vi "PSU_Command_Test.vi"() -> ()   [LabVIEW 2020]
uses:
  04db4537-6f8d-454a-96ee-4e1150a41387.vi
  0d439425-5a95-45a5-b8fa-685de4b41df2.vi
panel:
  in  "Stop":bool
  in  "Send":bool
  out "read buffer":string
  out "error out":errorcluster
  in  "write buffer":string
  out "Interface Description":string
  in  "Port":refnum<visa-resource-name>
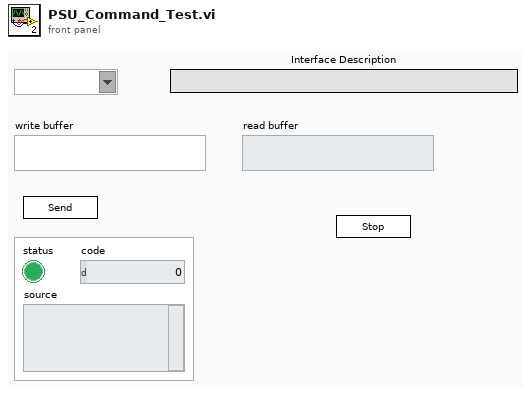
[diagram p1: front panel]
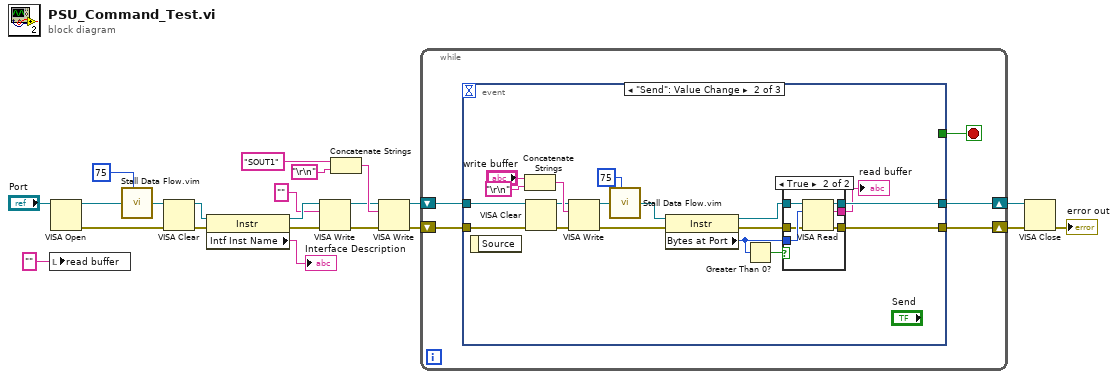
[diagram p0: block diagram]
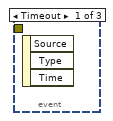
[diagram p2: hidden frame]
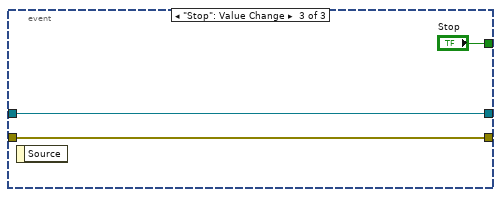
[diagram p4: hidden frame]
diagram:
  n1 = local write "read buffer"("" ("read buffer")) -> ()
  n2 = VISA Open(VISA resource name="Port") -> (VISA resource name=w5:refnum<visa-resource-name>, error out=w6:errorcluster)  [unwired: 4 in]
  n3 = call "Stall Data Flow.vim"("value in"=w5, "milliseconds to wait"=u32 75) -> ("value out"=w4:refnum<visa-resource-name>)  [unwired: 1 out]
  n4 = VISA Clear(VISA resource name=w4, error in (no error)=w6) -> (VISA resource name out=w3:refnum<visa-resource-name>, error out=w2:errorcluster)
  n5 = property class="Instr"(reference=w3, error in=w2) -> (reference out=w12:refnum<visa-resource-name>, error out=w10:errorcluster, "Intf Inst Name"=→"Interface Description":string)
  n6 = VISA Write(VISA resource name=w12, write buffer="", error in (no error)=w10) -> (VISA resource name out=w11:refnum<visa-resource-name>, error out=w9:errorcluster)  [unwired: 1 out]
  n7 = Concatenate Strings("SOUT1" ("string"), "\r\n") -> (w15:string)
  n8 = VISA Write(VISA resource name=w11, write buffer=w15, error in (no error)=w9) -> (VISA resource name out=w13:refnum<visa-resource-name>, error out=w14:errorcluster)  [unwired: 1 out]
  n9 = while {
    shift-right: [w26] -> w18
    shift-left: w14 -> [w24]
    shift-right: [w27] -> w19
    shift-left: w13 -> [w25]
    stop <- w23 stop-if-true
    n10 = event shown="[1] \"Send\": Value Change" {
      selector: _ -> [_ _ _]
      dyn-events: _ -> [_ _ _]
      timeout: _ -> [_ _ _]
      tunnel: w24 -> [_ w40 w54]
      tunnel: [_ w33 w55] -> w27
      tunnel: [_ w32 w54] -> w26
      tunnel: w25 -> [_ w42 w55]
      tunnel: [_ _ "Stop"] -> w23
      event Timeout {
        n11 = event-data() -> ()  [unwired: 1 in, 3 out]
      }
      event "Send": Value Change {
        n12 = event-data() -> ()  [unwired: 1 in, 1 out]
        n13 = Concatenate Strings("write buffer", "\r\n") -> (w43:string)
        n14 = VISA Clear(VISA resource name=w42, error in (no error)=w40) -> (VISA resource name out=w41:refnum<visa-resource-name>, error out=w39:errorcluster)
        n15 = VISA Write(VISA resource name=w41, write buffer=w43, error in (no error)=w39) -> (VISA resource name out=w31:refnum<visa-resource-name>, error out=w34:errorcluster)  [unwired: 1 out]
        n16 = call "Stall Data Flow.vim"("value in"=w31, "milliseconds to wait"=u32 75) -> ("value out"=w30:refnum<visa-resource-name>)  [unwired: 1 out]
        n17 = property class="Instr"(reference=w30, error in=w34) -> (reference out=w37:refnum<visa-resource-name>, error out=w38:errorcluster, "Bytes at Port"=w36:u32)
        n18 = Greater Than 0?(x=w36) -> (x > 0?=w35:bool)
        n19 = case shown="True" w35 {
          tunnel: w36 -> [_ w53]
          tunnel: w38 -> [w46 w52]
          tunnel: [w47 w51] -> w33
          tunnel: [w46 w50] -> w32
          tunnel: w37 -> [w47 w49]
          tunnel: [_ w48] -> w28
          frame False {
          }
          frame True {
            n20 = VISA Read(VISA resource name=w49, byte count=w53, error in (no error)=w52) -> (VISA resource name out=w51:refnum<visa-resource-name>, read buffer=w48:string, error out=w50:errorcluster)  [unwired: 1 out]
          }
        }
        "read buffer" <- w28
      }
      event "Stop": Value Change {
        n21 = event-data() -> ()  [unwired: 1 in, 1 out]
      }
    }
  }
  n22 = VISA Close(VISA resource name=w19, error in (no error)=w18) -> (error out=→"error out":errorcluster)
